vi "nirvififoEmulationRead.vi"(0 "In SCTL":bool, 1 "Ready for Output":bool, 4 "Timeout":i32, 5 "Width":i32=1024, 7 "ErrorIn":bool, 8 "Name":string="simul", 9 "Local? (F)":bool, 10 "Is Built-In FIFO?":bool, 13 "Is Handshake?":bool, 14 "Size":i32=1024, 15 "ref in wired":bool, 16 "Type":variant, 17 "Update Size?":bool) -> (21 "Element":variant, 24 "Empty":bool, 27 "Output Valid":bool)   [LabVIEW 2017]
uses:
  <instcachedir>/0/nirviFifoEmulationQueueMgr_E5CAEC123FF24DC58D834DCA3CDAA9B5.lvgen/nirviFifoEmulationQueueMgr_E5CAEC123FF24DC58D834DCA3CDAA9B5_000.vi
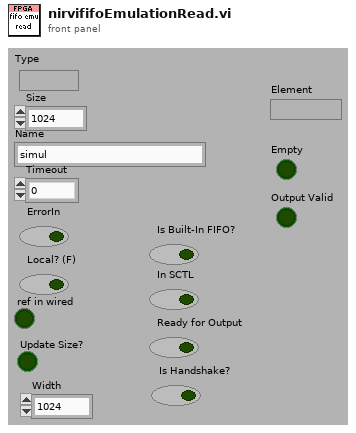
[diagram p1: front panel]
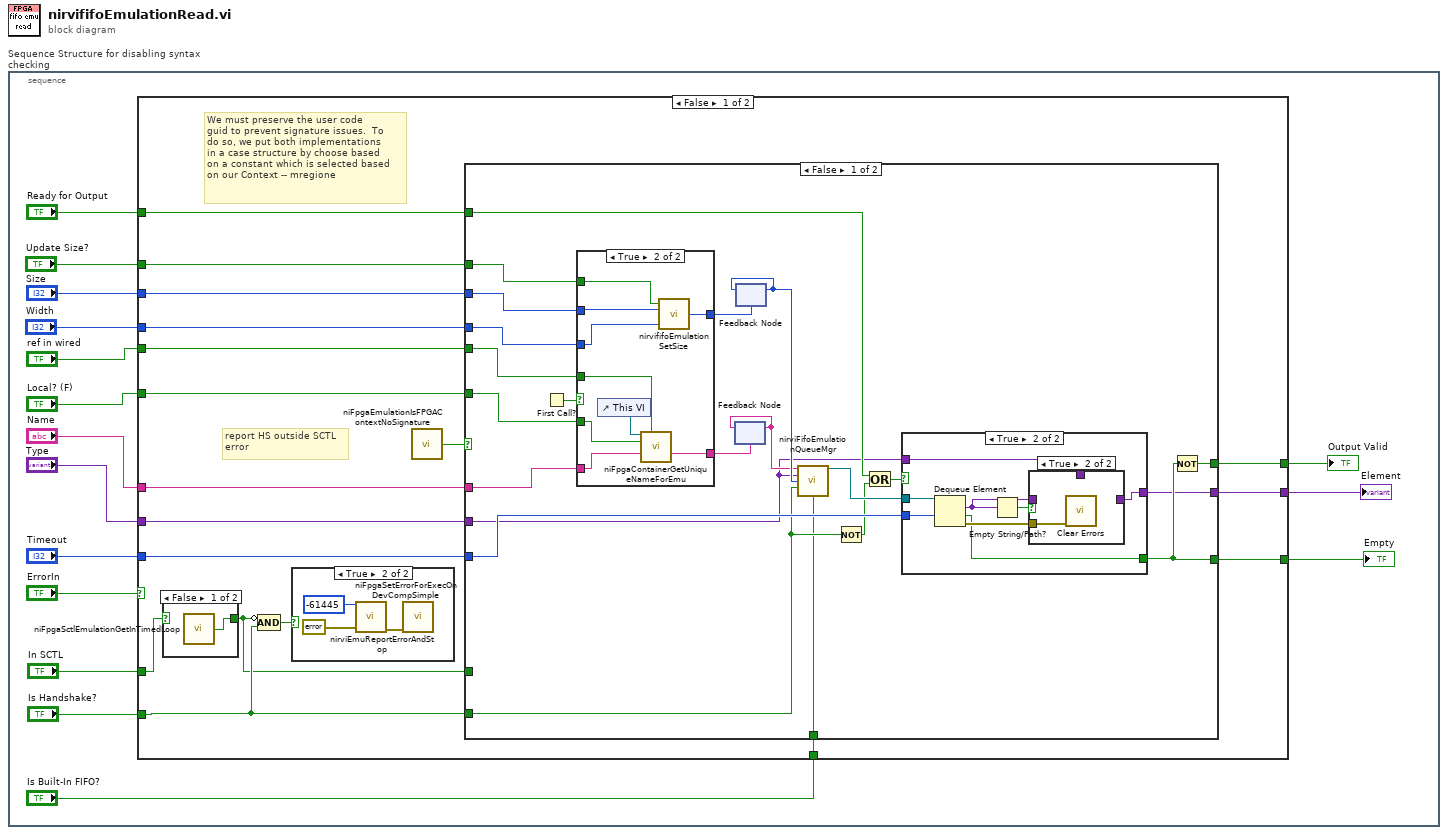
[diagram p0: block diagram]
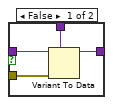
[diagram p5: hidden frame]
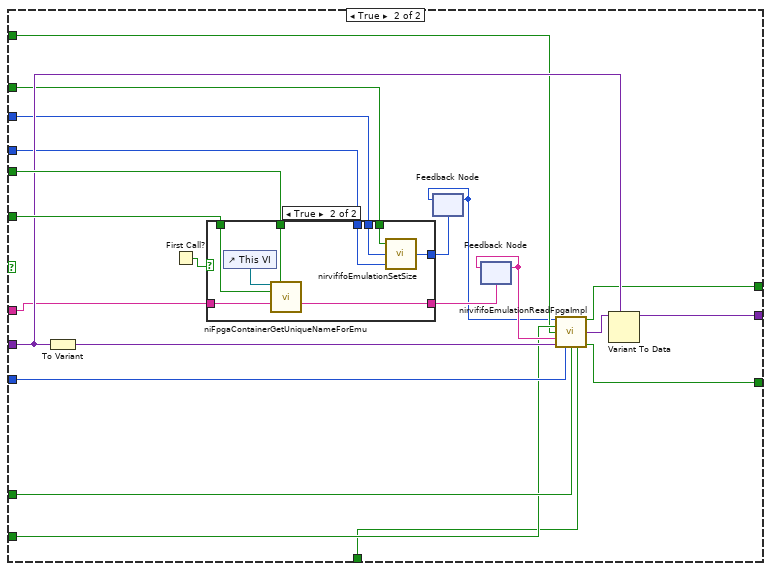
[diagram p7: hidden frame]
diagram:
  n1 = stacked-sequence "Sequence Structure for disabling syntax checking" {
    frame #0 {
      n2 = case shown="False" "ErrorIn" {
        tunnel: "Size" -> [w32 _]
        tunnel: "Name" -> [w29 _]
        tunnel: "Local? (F)" -> [w33 _]
        tunnel: "ref in wired" -> [w34 _]
        tunnel: [w31 _] -> w9
        tunnel: "In SCTL" -> [w20 _]
        tunnel: "Timeout" -> [w30 _]
        tunnel: [w28 w115] -> w7
        tunnel: "Type" -> [w27 w115]
        tunnel: "Update Size?" -> [w26 _]
        tunnel: "Width" -> [w25 _]
        tunnel: "Ready for Output" -> [w23 _]
        tunnel: "Is Handshake?" -> [w18 _]
        tunnel: [w22 _] -> w2
        tunnel: "Is Built-In FIFO?" -> [w21 _]
        frame False {
          # "report HS outside SCTL\nerror"
          # "We must preserve the user code\nguid to prevent signature issues.  To\ndo so, we put both implementations\nin a case structure by choose based\non a constant which is selected based\non our Context -- mregione"
          n3 = case shown="False" w20 {
            selector: w20 -> [_ w36]
            tunnel: [w35 w36] -> w17
            frame False {
              n4 = call <vilib>:"niFpgaSctlEmulationGetInTimedLoop.vi"() -> ("x != 0?"=w35:bool)  [unwired: 15 in]
            }
            frame True {
            }
          }
          n5 = Compound Arithmetic op=AND(invert w17, w18) -> (w19:bool)
          n6 = case shown="True" w19 {
            frame False {
            }
            frame True {
              n7 = call <vilib>:"niFpgaSetErrorForExecOnDevCompSimple.vi"("error code"=-61445, "error in"=errorcluster {"status"=FALSE, "code"=0, "source"=""}) -> ("error out"=w37:errorcluster)  [unwired: 13 in]
              n8 = call <vilib>:"nirviEmuReportErrorAndStop.vi"("error to report"=w37) -> ()  [unwired: 1 in, 14 out]
            }
          }
          n9 = call <vilib>:"niFpgaEmulationIsFPGAContextNoSignature.vi"() -> ("Is Fpga Context?"=w24:bool)  [unwired: 15 in]
          n10 = case shown="False" w24 {
            tunnel: w34 -> [w61 w98]
            tunnel: w33 -> [w60 w99]
            tunnel: w32 -> [w59 w89]
            tunnel: [w53 w97] -> w31
            tunnel: w17 -> [_ w100]
            tunnel: w30 -> [w58 w101]
            tunnel: w29 -> [w57 w85]
            tunnel: [w41 w95] -> w28
            tunnel: w27 -> [w40 w94]
            tunnel: w26 -> [w56 w90]
            tunnel: w25 -> [w55 w88]
            tunnel: w23 -> [w45 w92]
            tunnel: w18 -> [w44 w93]
            tunnel: [w54 w91] -> w22
            tunnel: w21 -> [w42 w84]
            frame False {
              n11 = First Call?() -> (First Call?: T/F=w52:bool)
              n12 = case shown="True" w52 {
                tunnel: w59 -> [_ w82]
                tunnel: w60 -> [_ w79]
                tunnel: w61 -> [_ w78]
                tunnel: w56 -> [_ w83]
                tunnel: w55 -> [_ w81]
                tunnel: [_ w76] -> w50
                tunnel: w57 -> [_ w77]
                tunnel: [_ w75] -> w51
                frame False {
                }
                frame True {
                  n13 = control-ref of="This VI"() -> (w80:refnum<vi>)
                  n14 = call <vilib>:"niFpgaContainerGetUniqueNameForEmu.vi"("parent VI"=w80, "ref in wired"=w78, "local"=w79, "name in"=w77) -> ("name out"=w76:string)  [unwired: 11 in]
                  n15 = call <vilib>:"nirvififoEmulationSetSize.vi"("width"=w81, "Size"=w82, "Update?"=w83) -> ("Actual Size"=w75:i32)
                }
              }
              n16 = feedback #1(w50) -> (w48:string)
              n17 = feedback-in #1(w48) -> ()
              n18 = feedback #2(w51) -> (w49:i32)
              n19 = feedback-in #2(w49) -> ()
              n20 = call-generic <vilib>:"nirviFifoEmulationQueueMgr.vi"("FIFO Name"=w48, "Element"=w40, "Size"=w49, "Is Handshake?"=w44, "Is Built-In FIFO?"=w42) -> ("FIFO"=w47:refnum<queue>)  [unwired: 10 in]
              n21 = Not(x=w44) -> (.not. x?=w43:bool)
              n22 = Or(x=w45, y=w43) -> (x .or. y?=w46:bool)
              n23 = case shown="True" w46 {
                tunnel: w58 -> [_ w69]
                tunnel: [_ w64] -> w53
                tunnel: w47 -> [_ w68]
                tunnel: [_ w66] -> w41
                tunnel: w40 -> [_ w65]
                frame False {
                }
                frame True {
                  n24 = Dequeue Element(queue=w68, timeout in ms (-1)=w69) -> (element=w62:variant, timed out?=w64:bool, error out=w67:errorcluster)  [unwired: 1 in, 1 out]
                  n25 = Empty String/Path?(string/path=w62) -> (empty?=w63:bool)
                  n26 = case shown="True" w63 {
                    tunnel: w67 -> [w73 w74]
                    tunnel: w62 -> [w72 _]
                    tunnel: [w71 _] -> w66
                    tunnel: w65 -> [w70 _]
                    frame False {
                      n27 = Variant To Data(error in=w73, type=w70, Variant=w72) -> (data=w71:variant)  [unwired: 1 out]
                    }
                    frame True {
                      n28 = call <vilib>:"Clear Errors.vi"("error in (no error)"=w74) -> ()  [unwired: 5 in, 2 out]
                    }
                  }
                }
              }
              n29 = Not(x=w53) -> (.not. x?=w54:bool)
            }
            frame True {
              n30 = To Variant(anything=w94) -> (Variant=w105:variant)
              n31 = First Call?() -> (First Call?: T/F=w104:bool)
              n32 = case shown="True" w104 {
                tunnel: w98 -> [_ w113]
                tunnel: w99 -> [_ w112]
                tunnel: [_ w111] -> w103
                tunnel: w90 -> [_ w110]
                tunnel: w89 -> [_ w109]
                tunnel: w88 -> [_ w108]
                tunnel: [_ w107] -> w87
                tunnel: w85 -> [_ w106]
                frame False {
                }
                frame True {
                  n33 = control-ref of="This VI"() -> (w114:refnum<vi>)
                  n34 = call <vilib>:"niFpgaContainerGetUniqueNameForEmu.vi"("parent VI"=w114, "ref in wired"=w113, "local"=w112, "name in"=w106) -> ("name out"=w111:string)  [unwired: 11 in]
                  n35 = call <vilib>:"nirvififoEmulationSetSize.vi"("width"=w108, "Size"=w109, "Update?"=w110) -> ("Actual Size"=w107:i32)
                }
              }
              n36 = feedback #3(w87) -> (w86:i32)
              n37 = feedback-in #3(w86) -> ()
              n38 = feedback #4(w103) -> (w102:string)
              n39 = feedback-in #4(w102) -> ()
              n40 = call <vilib>:"nirvififoEmulationReadFpgaImpl.vi"("Size"=w86, "Is Handshake?"=w93, "Ready for Output?"=w92, "Name"=w102, "Init Val"=w105, "Timeout"=w101, "In Sctl?"=w100, "Is Built-In FIFO?"=w84) -> ("Output Valid?"=w91:bool, "Data Out"=w96:variant, "Empty?"=w97:bool)  [unwired: 5 in]
              n41 = Variant To Data(type=w94, Variant=w96) -> (data=w95:variant)  [unwired: 1 in, 1 out]
            }
          }
        }
        frame True {
        }
      }
      "Element" <- w7
      "Empty" <- w9
      "Output Valid" <- w2
    }
  }
